vi "DG Control.vi"() -> ()   [LabVIEW 2017]
uses:
  <instrlib>/tio-labview/TIO Library/TIO Stream Open.vi
  <instrlib>/tio-labview/TIO Library/TIO RPC Send REQuest.vi
  <vilib>/Utility/error.llb/Clear Errors.vi
  <instrlib>/tio-labview/TIO Library/TIO RPC Parse Reply.vi
  <instrlib>/tio-labview/TIO Library/TIO RPC Parse Reply Error.vi
  <instrlib>/tio-labview/TIO Library/TIO Data Stream Parse timebase Info.vi
  <instrlib>/tio-labview/TIO Library/TIO Data Stream Parse pstream Info.vi
  <instrlib>/tio-labview/TIO Library/TIO Data Stream Parse dstream Info.vi
  <vilib>/Utility/High Resolution Relative Seconds.vi
  <instrlib>/tio-labview/TIO Library/TIO Serial Port Name Search.vi
  <instrlib>/tio-labview/TIO Library/TIO Stream Write.vi
  <instrlib>/tio-labview/TIO Library/TIO RPC Form Request.vi
  <instrlib>/tio-labview/TIO Library/TIO SLIP Serial Write.vi
  <instrlib>/tio-labview/TIO Library/TIO Form Packet.vi
  <instrlib>/tio-labview/TIO Library/TIO SLIP Encode.vi
  <instrlib>/tio-labview/TIO Library/TIO Serial Checksum CRC32.vi
  <vilib>/Utility/tcp.llb/UDP Multicast Open.vi
  <vilib>/Utility/tcp.llb/UDP Multicast Read-Write Open.vi
  <instrlib>/tio-labview/TIO Library/TIO Serial Port Discovery.vi
  <vilib>/Instr/_visa.llb/VISA Configure Serial Port (Instr).vi
  <instrlib>/tio-labview/TIO Library/TIO RPC Blocking.vi
  <instrlib>/tio-labview/TIO Library/TIO Stream Read Non-blocking.vi
  <instrlib>/tio-labview/TIO Library/TIO RPC Send Heartbeat.vi
panel:
  out "Status":T1(ring)
  out "Load":dbl[unit]=1.0 format="%#_3g"
  in  "Abort":bool
  in  "Save":bool
  in  "Waveform Frequency":dbl[unit]=10.0
  in  "Degauss":bool
  in  "Waveform Current":dbl[unit]=1.0
  in  "Waveform Length":dbl[unit]=100.0
  in  "Reset":bool
  in  "URL":refnum<visa-resource-name>="tcp://localhost"
  in  "Quit":bool
  in  "Plot Duration":dbl[unit]=200.0
  out "A":T2(graph)
  out "B":T2(graph)
  out "XY Graph":cluster{"Timeseries":dbl[], "Timeseries":dbl[]}(graph)
  out "ID":string
  # "DG"
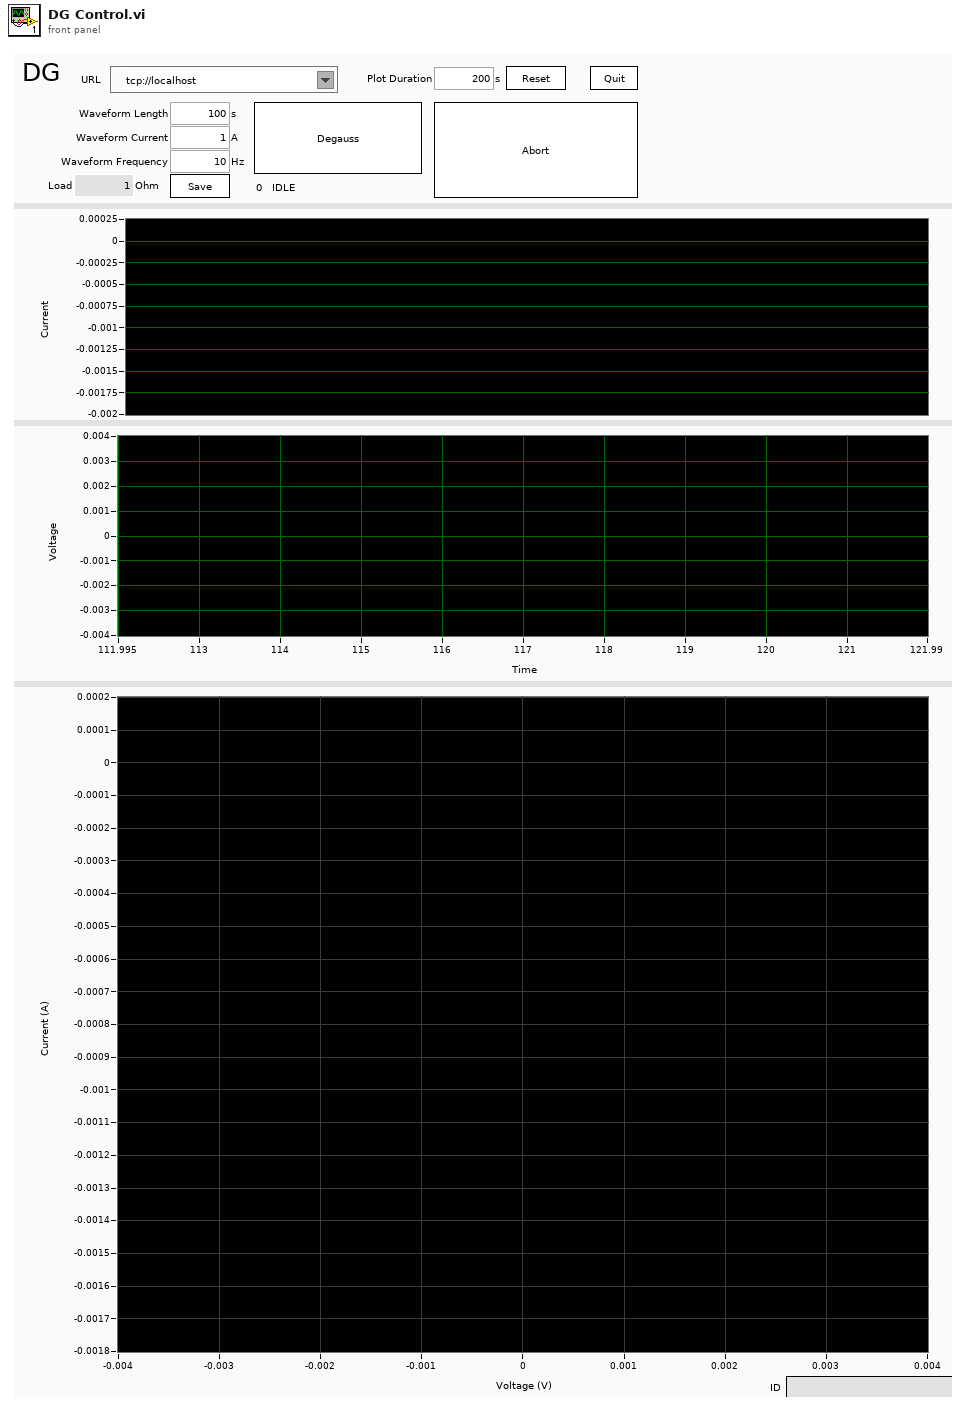
[diagram p1: front panel]
types:
  T1 = enum16{"IDLE", "ERROR LOAD", "ERROR OFFSET", "STARTING", "CALIBRATING OFFSET", "CALIBRATING LOAD", "SOAK", "RUNNING"}
  T2 = cluster{"start":dbl, "dt":dbl, "Timeseries":dbl[]}
  T3 = cluster{"TS Connection":cluster{"Type":enum16{"Serial", "TCP", "UDP", "mUDP"}, "URL":refnum<visa-resource-name>, "TO":u32, "Addr":u32, "Port":i32, "TCP":refnum<k5>, "UDP":refnum<k16>, "Route":string}, "REQ":refnum<queue>, "REP":refnum<queue>}
  T4 = cluster{"start":dbl, "dt":dbl, "Timeseries":sgl[][]}
  T5 = cluster{"Awaiting REP":bool, "REQ ID":u32, "streams in":cluster{"id":u16, "timebase id":u16, "period":u32, "offset":u32, "sample number":u64, "total components":u16, "flags":u16, "components":cluster{"source id":u16, "flags":u16, "period":u32, "offset":u32}[]}[], "sources":cluster{"id":u16, "timebase_id":u16, "period":u32, "offset":u32, "fmt":i32, "flags":u16, "channels":u16, "type":u8, "name":string, "column names":string[], "title":string, "units":string}[], "timebases":cluster{"id":u16, "source":u8, "epoch":u8, "start time":u64, "period numerator (µs)":u32, "period denominator (µs)":u32, "flags":u32, "stability":sgl, "source id":string}[]}
  T6 = cluster{"stream ID":u16, "Sample Number":u32, "Raw Data":string}
  T7 = cluster{"TC Connection":cluster{"Type":enum16{"Serial", "TCP", "UDP", "mUDP"}, "URL":refnum<visa-resource-name>, "TO":u32, "Addr":u32, "Port":i32, "TCP":refnum<k5>, "UDP":refnum<k16>, "Route":string}, "REQ":refnum<queue>, "REP":refnum<queue>}
  T8 = cluster{"start":dbl, "dt":dbl, "Timeseries":dbl[][]}
  T9 = cluster{"Name":string, "Waveform":cluster{"start":dbl, "dt":dbl, "Timeseries":dbl[][]}}[]
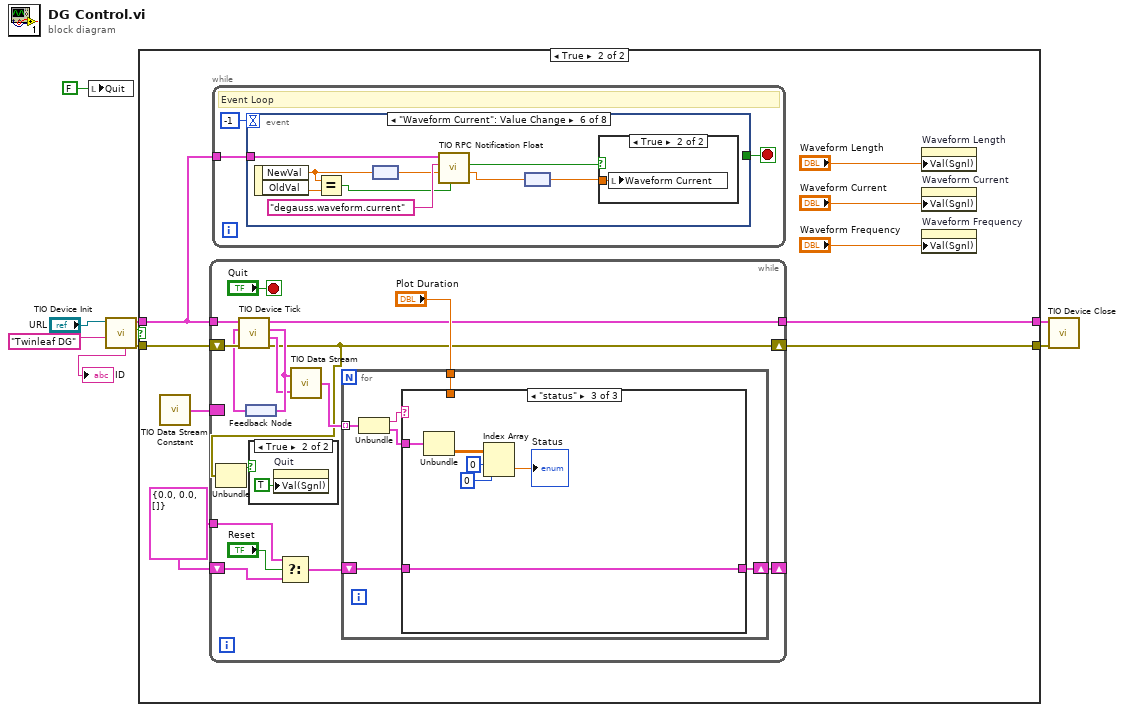
[diagram p0: block diagram]
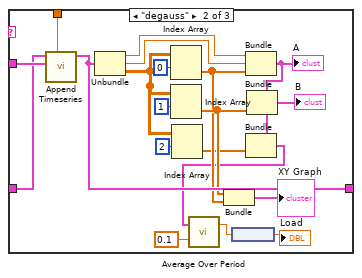
[diagram p5: hidden frame]
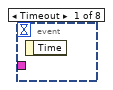
[diagram p6: hidden frame]
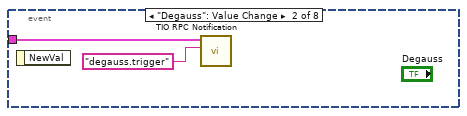
[diagram p7: hidden frame]
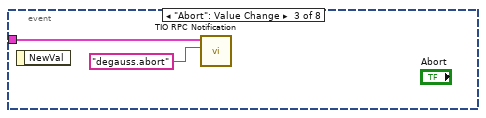
[diagram p8: hidden frame]
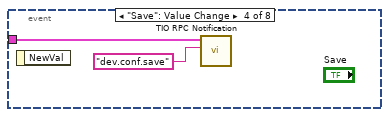
[diagram p9: hidden frame]
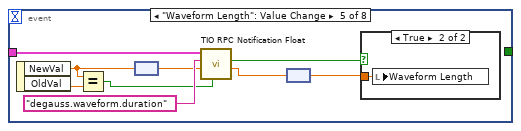
[diagram p10: hidden frame]
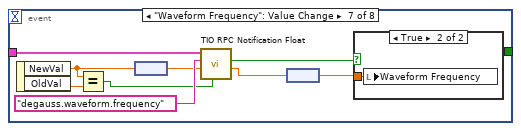
[diagram p13: hidden frame]
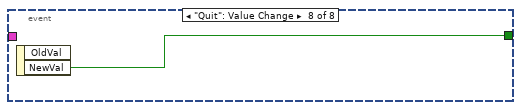
[diagram p15: hidden frame]
diagram:
  n1 = local write "Quit"(FALSE ("Kill")) -> ()
  n2 = call <instrlib>:"TIO Device Init.vi"("ID"="Twinleaf DG" ("Prefix"), "URL"="URL") -> ("error out"=w8:errorcluster, 2:"ID Verified"=w4:bool, "TIO"=w9:T3, 4:"ID Verified"=→"ID":string)  [unwired: 5 in, 1 out]
  n3 = case shown="True" w4 {
    tunnel: w9 -> [w11 w19]
    tunnel: w8 -> [w10 w20]
    tunnel: [w10 w14] -> w3
    tunnel: [w11 w13] -> w2
    frame False {
    }
    frame True {
      w12 = T4 {"start"=0.0, "dt"=0.0, "Timeseries"=[]}
      n4 = call <instrlib>:"TIO Data Stream Constant.vi"() -> ("TIO State"=w18:T5)
      n5 = while {
        tunnel: w19 -> [w36]
        shift-right: [w32] -> _
        shift-left: w12 -> [w24]
        border: w18 -> [_]
        tunnel: [w27] -> w13
        tunnel: w12 -> [w25]
        shift-right: [w22] -> w14
        shift-left: w20 -> [w35]
        stop <- "Quit" stop-if-true
        n6 = feedback #1() -> (w31:T5)
        n7 = call <instrlib>:"TIO Device Tick.vi"("Error in"=w35, "TIO State"=w31, "TIO"=w36) -> ("Error out"=w22:errorcluster, "Data Out"=w28:T6, "TIO State"=w29:T5, "TIO"=w27:T7)  [unwired: 5 in]
        n8 = Unbundle(w22) -> ("status"=w21:bool)  [unwired: 2 out]
        n9 = feedback-in #1(w29) -> ()
        n10 = case shown="True" w21 {
          frame False {
          }
          frame True {
            n11 = property on="Quit" class="Bool (strict)"("Val(Sgnl)"=TRUE ("Value (Signaling)")) -> ()  [unwired: 2 in, 2 out]
          }
        }
        n12 = Select(t=w25, s="Reset", f=w24) -> (s? t:f=w23:T8)
        n13 = call <instrlib>:"TIO Data Stream.vi"("Raw Data"=w28, "TIO State"=w29) -> ("Data Out"=w30:T9)
        n14 = for {
          tunnel: "Plot Duration" -> [w43]
          tunnel: w30 -> [w40] mode=indexing
          shift-right: [w42] -> w32
          shift-left: w23 -> [w41]
          n15 = Unbundle(w40) -> ("Name"=w39:string, "Waveform"=w38:T8)
          n16 = case shown="\"status\"" w39 {
            tunnel: w43 -> [_ w64 _]
            tunnel: w38 -> [_ w58 w67]
            tunnel: [w44 w57 w68] -> w42
            tunnel: w41 -> [w44 w56 w68]
            frame Default {
            }
            frame "degauss" {
              n17 = call <instrlib>:"Append Timeseries.vi"("Duration"=w64, "In New"=w58, "In Old"=w56) -> ("Appended"=w57:T8)  [unwired: 8 in]
              n18 = Unbundle(w57) -> ("start"=w63:dbl, "dt"=w59:dbl, "Timeseries"=w51:dbl[][])
              n19 = Index Array(array=w51, index (row)=0 ("disabled index (col)")) -> (element=w53:dbl[])  [unwired: 1 in]
              n20 = Index Array(array=w51, index (row)=1 ("disabled index (col)")) -> (element=w54:dbl[])  [unwired: 1 in]
              n21 = Index Array(array=w51, index (row)=2 ("disabled index (col)")) -> (element=w46:dbl[])  [unwired: 1 in]
              n22 = Bundle("Timeseries"=w54, "Timeseries"=w53) -> (→"XY Graph":cluster{"Timeseries":dbl[], "Timeseries":dbl[]})  [unwired: 1 in]
              n23 = Bundle("start"=w63, "dt"=w59, "Timeseries"=w53) -> (w47:T2)  [unwired: 1 in]
              "A" <- w47
              n24 = Bundle(cluster=w47, "Timeseries"=w46) -> (w45:T2)  [unwired: 2 in]
              n25 = call <instrlib>:"Average Over Period.vi"("Average Period"=dbl[unit] 0.1 ("Period"), "Waveform"=w45) -> ("Average"=w49:dbl)  [unwired: 1 in]
              n26 = node(w49) -> (→"Load":dbl[unit])
              n27 = Bundle(cluster=w47, "Timeseries"=w54) -> (→"B":T2)  [unwired: 2 in]
            }
            frame "status" {
              n28 = Unbundle(w67) -> ("Timeseries"=w69:dbl[][])  [unwired: 2 out]
              n29 = Index Array(array=w69, index (row)=0 ("disabled index (col)"), index (col)=0 ("disabled index (col)")) -> (element=→"Status":dbl)
            }
          }
        }
      }
      n30 = while {
        tunnel: w19 -> [w72]
        stop <- w71 stop-if-true
        # "Event Loop"
        n31 = event shown="[5] \"Waveform Current\": Value Change" {
          selector: _ -> [_ _ _ _ _ _ _ _]
          dyn-events: _ -> [_ _ _ _ _ _ _ _]
          timeout: -1 -> [_ _ _ _ _ _ _ _]
          tunnel: w72 -> [_ w75 w77 w79 w88 w98 w108 _]
          tunnel: [_ _ _ _ _ _ _ w110] -> w71
          event Timeout {
            n32 = event-data() -> ()  [unwired: 1 in, 1 out]
          }
          event "Degauss": Value Change {
            n33 = event-data() -> ()  [unwired: 1 in, 1 out]
            n34 = call <instrlib>:"TIO RPC Notification.vi"("Topic"="degauss.trigger", "TIO"=w75) -> ()  [unwired: 6 in, 3 out]
          }
          event "Abort": Value Change {
            n35 = event-data() -> ()  [unwired: 1 in, 1 out]
            n36 = call <instrlib>:"TIO RPC Notification.vi"("Topic"="degauss.abort", "TIO"=w77) -> ()  [unwired: 6 in, 3 out]
          }
          event "Save": Value Change {
            n37 = event-data() -> ()  [unwired: 1 in, 1 out]
            n38 = call <instrlib>:"TIO RPC Notification.vi"("Topic"="dev.conf.save", "TIO"=w79) -> ()  [unwired: 6 in, 3 out]
          }
          event "Waveform Length": Value Change {
            n39 = event-data() -> ("NewVal"=w85:dbl[unit], "OldVal"=w87:dbl[unit])  [unwired: 1 in]
            n40 = Equal?(x=w85, y=w87) -> (x = y?=w83:bool)
            n41 = node(w85) -> (w84:dbl)
            n42 = call <instrlib>:"TIO RPC Notification Float.vi"("Read"=w83, "Set value"=w84, "Topic"="degauss.waveform.duration", "TIO"=w88) -> ("Get value (default if error)"=w81:sgl, "Response"=w82:bool)  [unwired: 4 in, 1 out]
            n43 = node(w81) -> (w80:sgl[unit])
            n44 = case shown="True" w82 {
              tunnel: w80 -> [_ w89]
              frame False {
              }
              frame True {
                n45 = local write "Waveform Length"(w89) -> ()
              }
            }
          }
          event "Waveform Current": Value Change {
            n46 = event-data() -> ("NewVal"=w95:dbl[unit], "OldVal"=w97:dbl[unit])  [unwired: 1 in]
            n47 = Equal?(x=w95, y=w97) -> (x = y?=w93:bool)
            n48 = node(w95) -> (w94:dbl)
            n49 = call <instrlib>:"TIO RPC Notification Float.vi"("Read"=w93, "Set value"=w94, "Topic"="degauss.waveform.current", "TIO"=w98) -> ("Get value (default if error)"=w91:sgl, "Response"=w92:bool)  [unwired: 4 in, 1 out]
            n50 = node(w91) -> (w90:sgl[unit])
            n51 = case shown="True" w92 {
              tunnel: w90 -> [_ w99]
              frame False {
              }
              frame True {
                n52 = local write "Waveform Current"(w99) -> ()
              }
            }
          }
          event "Waveform Frequency": Value Change {
            n53 = event-data() -> ("NewVal"=w105:dbl[unit], "OldVal"=w107:dbl[unit])  [unwired: 1 in]
            n54 = Equal?(x=w105, y=w107) -> (x = y?=w103:bool)
            n55 = node(w105) -> (w104:dbl)
            n56 = call <instrlib>:"TIO RPC Notification Float.vi"("Read"=w103, "Set value"=w104, "Topic"="degauss.waveform.frequency", "TIO"=w108) -> ("Get value (default if error)"=w101:sgl, "Response"=w102:bool)  [unwired: 4 in, 1 out]
            n57 = node(w101) -> (w100:sgl[unit])
            n58 = case shown="True" w102 {
              tunnel: w100 -> [_ w109]
              frame False {
              }
              frame True {
                n59 = local write "Waveform Frequency"(w109) -> ()
              }
            }
          }
          event "Quit": Value Change {
            n60 = event-data() -> ("NewVal"=w110:bool)  [unwired: 1 in, 1 out]
          }
        }
      }
      n61 = property on="Waveform Length" class="DigNum (strict)"("Val(Sgnl)"="Waveform Length") -> ()  [unwired: 2 in, 2 out]
      n62 = property on="Waveform Current" class="DigNum (strict)"("Val(Sgnl)"="Waveform Current") -> ()  [unwired: 2 in, 2 out]
      n63 = property on="Waveform Frequency" class="DigNum (strict)"("Val(Sgnl)"="Waveform Frequency") -> ()  [unwired: 2 in, 2 out]
    }
  }
  n64 = call <instrlib>:"TIO Device Close.vi"("Error in"=w3, "TIO"=w2) -> ()  [unwired: 10 in]
